vi "thcd_test.vi"() -> ()   [LabVIEW 2013]
uses:
  thcd_controls/ctrl_chn_thcd.ctl
  thcd_controls/ctrl_uom_thcd.ctl
  thcd_controls/ctrl_gid_thcd.ctl
  thcd_commands/thcd_set_uom.vi
  thcd_commands/thcd_get_samp.vi
panel:
  out "thcd_res 2":dbl
  in  "thcd_com 2":T1(ring)
  in  "thcd_val 3":T2
  in  "thcd_val 2":T3
  out "thcd_st 3":bool
  out "thcd_res_msg 2":string
  in  "thcd_com":T1(ring)
  in  "thcd_val":dbl min=0.0 max=99999.0 format="%#.6g"
  in  "Serial Settings:Baud Rate":u32(ring)=19200 items=["9.6KHz"=9600, "19.2KHz"=19200]
  in  "thcd_visa":refnum<visa-resource-name>
  out "thcd_res":T5
  out "res_4":T6
  out "thcd_st 2":bool
  out "error out":errorcluster
  out "thcd_res_str 2":string
  out "thcd_st":bool
  out "thcd_res_str":string="\r"
  out "thcd_res_msg":string
  in  "thcd_ch":T4=enum."1"
  in  "thcd_b2r":u32
  in  "thcd_delay":u32=500
  # "GETTERS"
  # "SETTERS"
  # "STAT and READ ALL"
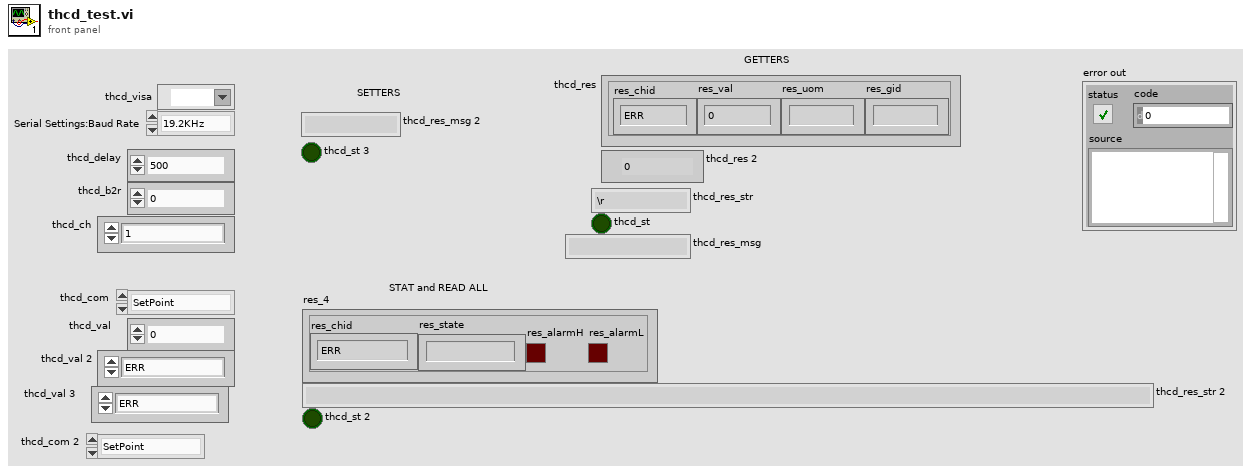
[diagram p1: front panel]
types:
  T1 = enum16{"SetPoint", "AlarmH", "AlarmL", "Multiplier", "CalibValue"}
  T2 = typedef "ctrl_gid_thcd.ctl" = enum16{"ERR", "1", "2", "C3H6O_1", "C2H3N", "C2H2", "Air", "C3H4_1", "NH3", "Ar", "AsH3", "C6H6", "BCl3", "BF3", "Br2", "15", "16", "CBrF3", "C4H10_1", "19", "C4H8_1", "CO2", "CS2", "CO", "CCl4", "COS", "Cl2", "ClF3", "28", "29", "CHCl3", "31", "32", "C4H8_2", "C2N2", "ClCN", "C4H8_3", "C3H6", "H22", "B2H6", "40", "R21", "42", "43", "44", "45", "46", "47", "48", "C2H7N_1", "C2H6O_1", "C2H6S_1", "C4H6_1", "C2H6", "54", "55", "C2H6O_2", "C4H6_2", "C2H7N_2", "C8H10", "60", "61", "C2H5F", "C2H4", "64", "65", "C2H4O", "C2H4N", "68", "C2H6S_2", "F2", "CH2O", "CCl3F", "73", "CClF3", "CF4", "76", "CHF3", "78", "C4H4O", "He", "C3HF7", "HMDS", "83", "C6H14", "C6F6", "C6H12_1", "N2H4", "H2", "HBr", "HCl", "CHN", "HF", "HI", "H2Se", "H2S", "C4H10_2", "97", "C4H8_4", "C5H12_1", "C3H8O_1", "101", "C2H2O", "Kr", "CH4", "CH4O", "106", "C3H4_2", "CH5N", "CH3Br", "CH3Cl", "C7H14", "C3H9N", "C3H8O_2", "C3H8S", "CH3F", "116", "CH3I", "CH4S", "C6H12_2", "C3H6O_2", "Ne", "NO", "N2", "NO2", "N2O4", "NF3", "127", "NOCl", "N2O", "C5H12_2", "C8H18", "O2", "F2O", "O3", "B5H9", ""}
  T3 = typedef "ctrl_uom_thcd.ctl" = enum16{"ERR", "SCCM", "SLM", "%", "V", "MV", "CNT", "NLM", "SLS", "NLS", "SLH", "NLH", "SMLM", "NMLM", "SMLS", "NMLS", "SMLH", "NMLH", "NCCM", "SCCS", "NCCS", "SCCH", "NCCH", "SCFM", "NCFM", "SCFS", "NCFS", "SCFH", "NCFH", "SCMM", "NCMM", "SCMS", "NCMS", "SCMH", "NCMH", "SCIM", "NCIM", "SCIS", "NCIS", "SCIH", "NCIH", "LBM", "LBS", "LBH", "KgM", "KgS", "KgH", "GRM", "GMS", "GRH", "MolM", "MolS", "MolH", "KMolM", "KMolS", "KMolH", "W", "BPS", "Sec", "Min", "Hrs", "WH", "Torr", "Bar", "Pa", "inH2O", "PSIA", "PSIG"}
  T4 = typedef "ctrl_chn_thcd.ctl" = enum8{"ERR", "1", "2", "3", "4"}
  T5 = cluster{"res_chid":T4, "res_val":dbl, "res_uom":string, "res_gid":string}
  T6 = cluster{"res_chid":T4, "res_state":string, "res_alarmH":bool, "res_alarmL":bool}
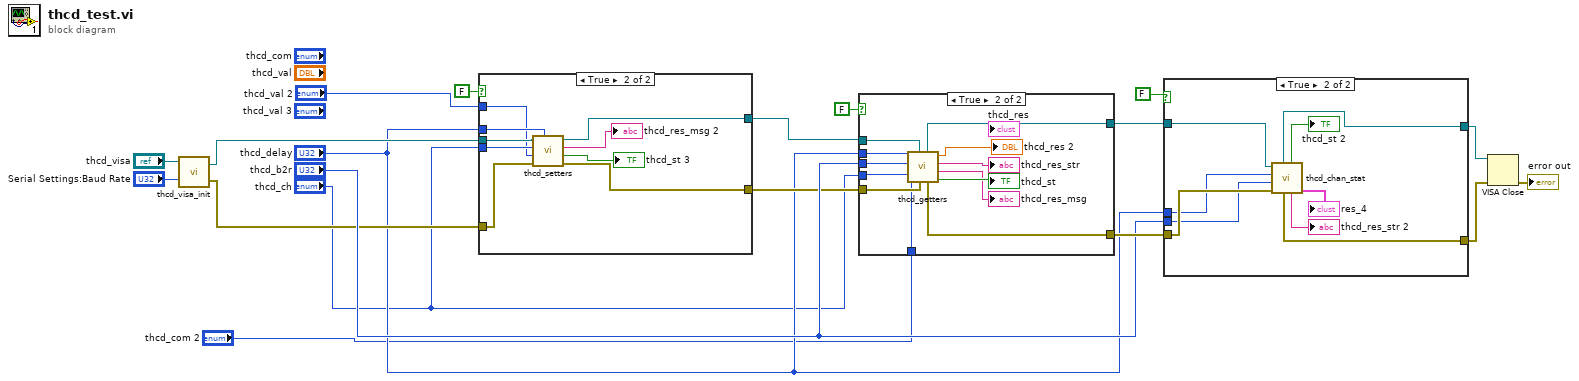
[diagram p0: block diagram]
diagram:
  n1 = call "thcd_visa_init.vi"("Serial Settings:Baud Rate"="Serial Settings:Baud Rate", "thcd_visa"="thcd_visa") -> ("err_out"=w7:errorcluster, "thcd_visa"=w9:refnum<visa-resource-name>)  [unwired: 1 in]
  n2 = case shown="True" FALSE {
    tunnel: w9 -> [w21 w30]
    tunnel: [w21 w29] -> w8
    tunnel: w7 -> [w20 w28]
    tunnel: [w20 w27] -> w6
    tunnel: "thcd_delay" -> [_ w26]
    tunnel: "thcd_ch" -> [_ w25]
    tunnel: "thcd_val 2" -> [_ w22]
    frame False {
    }
    frame True {
      n3 = call-poly "thcd_setters.vi"("thcd_delay"=w26, "err_in"=w28, "thcd_val"=w22, "thcd_ch"=w25, "thcd_visa"=w30) -> ("err_out"=w27:errorcluster, "thcd_st"=→"thcd_st 3":bool, "thcd_res_msg"=→"thcd_res_msg 2":string, "thcd_visa"=w29:refnum<visa-resource-name>)  [unwired: 1 in]
    }
  }
  n4 = case shown="True" FALSE {
    tunnel: [w32 w42] -> w19
    tunnel: [w31 w41] -> w18
    tunnel: "thcd_delay" -> [_ w40]
    tunnel: "thcd_b2r" -> [_ w39]
    tunnel: "thcd_ch" -> [_ w38]
    tunnel: w8 -> [w32 w37]
    tunnel: w6 -> [w31 w36]
    tunnel: "thcd_com 2" -> [_ w35]
    frame False {
    }
    frame True {
      n5 = call-poly "thcd_getters.vi"("err_in"=w36, "thcd_visa"=w37, "thcd_com"=w35, "thcd_ch"=w38, "thcd_b2r"=w39, "thcd_delay"=w40) -> ("thcd_st"=→"thcd_st":bool, "thcd_res_msg"=→"thcd_res_msg":string, "thcd_res_str"=→"thcd_res_str":string, "thcd_res"=→"thcd_res 2":dbl, "err_out"=w41:errorcluster, "thcd_visa"=w42:refnum<visa-resource-name>)
    }
  }
  n6 = case shown="True" FALSE {
    tunnel: w19 -> [w45 w55]
    tunnel: w18 -> [w46 w54]
    tunnel: "thcd_delay" -> [_ w53]
    tunnel: "thcd_b2r" -> [_ w52]
    tunnel: [w45 w51] -> w16
    tunnel: [w46 w50] -> w15
    frame False {
    }
    frame True {
      n7 = call "thcd_chan_stat.vi"("err_in"=w54, "thcd_b2r"=w52, "thcd_delay"=w53, "thcd_visa"=w55) -> ("thcd_res_4"=→"res_4":T6, "thcd_res_str"=→"thcd_res_str 2":string, "thcd_st"=→"thcd_st 2":bool, "err_out"=w50:errorcluster, "thcd_visa"=w51:refnum<visa-resource-name>)  [unwired: 3 out]
    }
  }
  n8 = VISA Close(VISA resource name=w16, error in (no error)=w15) -> (error out=→"error out":errorcluster)
